vi "PSFL1dll.vi"(8 "error in (no error)":errorcluster, 11 "Inputs":T2) -> (0 "error out":errorcluster, 3 "Outputs":T1)   [LabVIEW 2015]
doc: "SINGLE-PHASE FLASH SUBROUTINES\n\nsubroutine PSFL1dll(p, s, z, kph, t, d, ierr, herr, herr_length)\n\nThese routines accept only single-phase states as inputs. They will be\nfaster than the corresponding general routines, but will fail if called\nwith an incorrect phase specification. The phase-specific subroutines\nalso do not check limits, so may fail if called outside the range of the\nequation of state. The following single-phase routines are available.\n\nINPUTS: \np -- pressure [kPa]\ns -- entropy [[J/mol-K]\nz -- overall (bulk) composition [array of mol frac]\nkph -- phase flag: 1 = liquid\n 2 = vapor\nt -- temperature [K]\nd -- molar density [mol/L]\n\nOUTPUTS:\nt -- temperature [K] (present only for HSFL1)\nd -- molar density [mol/L]\nierr -- error flag: 0 = successful\nherr -- error string (character*255 variable if ierr<>0)\nherr_length -- length of variable herr (default: 255)"
uses:
  REFPROP.dll
panel:
  # "REFPROP-PSFL1dll.vi"
  # "void  PSFL1dll(double *p, double *s, double *z, int32_t *kph, double *t, double *d, int32_t *ierr, CStr herr, int32_t herr_length);"
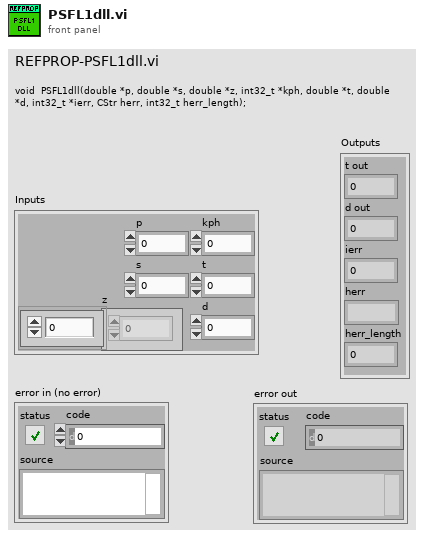
[diagram p1: front panel]
types:
  T1 = cluster{"t out":dbl, "d out":dbl, "ierr":i32, "herr":string, "herr_length":i32}
  T2 = cluster{"p":dbl, "s":dbl, "z":dbl[], "kph":i32, "t":dbl, "d":dbl}
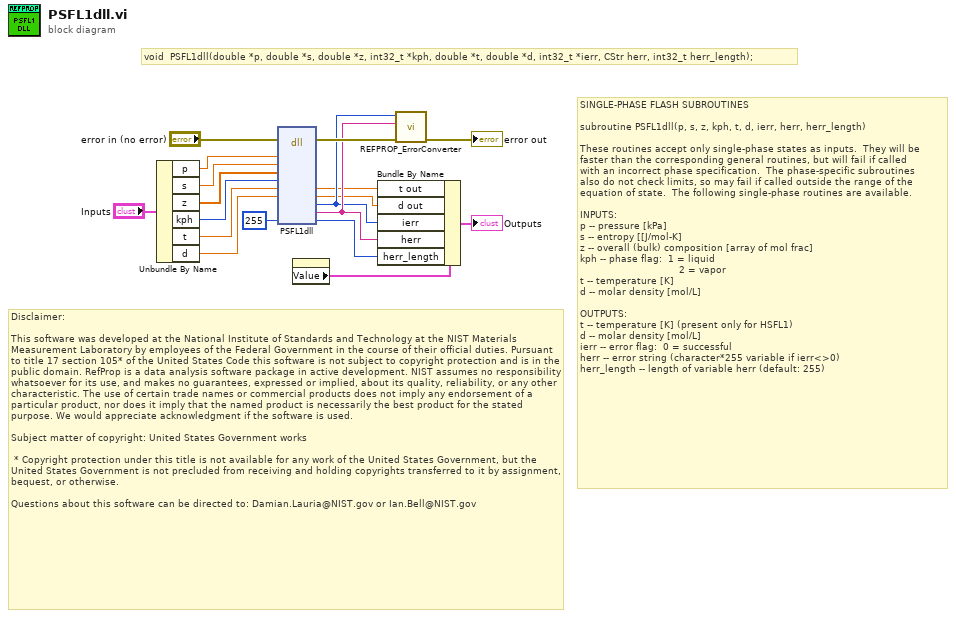
[diagram p0: block diagram]
diagram:
  # "Disclaimer:\n\nThis software was developed at the National Institute of Standards and Technology at the NIST Materials Measurement Laboratory by employees of the Federal Government in the course of their official duties. Pursuant to title 17 section 105* of the United States Code this software is not subject to copyright protection and is in the public domain. RefProp is a data analysis software package in active development. NIST assumes no responsibility whatsoever for its use, and makes no guarantees, expressed or implied, about its quality, reliability, or any other characteristic. The use of certain trade names or commercial products does not imply any endorsement of a particular product, nor does it imply that the named product is necessarily the best product for the stated purpose. We would appreciate acknowledgment if the software is used.\n \nSubject matter of copyright: United States Government works\n  \n * Copyright protection under this title is not available for any work of the United States Government, but the United States Government is not precluded from receiving and holding copyrights transferred to it by assignment, bequest, or otherwise.\n\nQuestions about this software can be directed to: Damian.Lauria@NIST.gov or Ian.Bell@NIST.gov"
  # "void  PSFL1dll(double *p, double *s, double *z, int32_t *kph, double *t, double *d, int32_t *ierr, CStr herr, int32_t herr_length);"
  # "SINGLE-PHASE FLASH SUBROUTINES\n\nsubroutine PSFL1dll(p, s, z, kph, t, d, ierr, herr, herr_length)\n\nThese routines accept only single-phase states as inputs.  They will be\nfaster than the corresponding general routines, but will fail if called\nwith an incorrect phase specification.  The phase-specific subroutines\nalso do not check limits, so may fail if called outside the range of the\nequation of state.  The following single-phase routines are available.\n\nINPUTS: \np -- pressure [kPa]\ns -- entropy [[J/mol-K]\nz -- overall (bulk) composition [array of mol frac]\nkph -- phase flag:  1 = liquid\n                                 2 = vapor\nt -- temperature [K]\nd -- molar density [mol/L]\n\nOUTPUTS:\nt -- temperature [K] (present only for HSFL1)\nd -- molar density [mol/L]\nierr -- error flag:  0 = successful\nherr -- error string (character*255 variable if ierr<>0)\nherr_length -- length of variable herr (default: 255)"
  n1 = Unbundle By Name("Inputs") -> ("p"=w6:dbl, "s"=w5:dbl, "z"=w4:dbl[], "kph"=w3:i32, "t"=w2:dbl, "d"=w1:dbl)
  n2 = dll-call lib="C:/Users/lauria/Desktop/REFPROP 10 LabVIEW Wrapper BETA/REFPROP/REFPROP.*" fn="PSFL1dll"(error in="error in (no error)", "p"=w6, "s"=w5, "z"=w4, "kph"=w3, "t"=w2, "d"=w1, "herr_length"=255) -> (error out=w18:errorcluster, "t"=w8:dbl, "d"=w9:dbl, "ierr"=w10:i32, "herr"=w11:string, "herr_length"=w12:i32)  [unwired: 9 in, 1 out]
  n3 = property on="Outputs" class="Clust (strict)"() -> ("Value"=w14:T1)  [unwired: 2 in, 2 out]
  n4 = Bundle By Name(cluster=w14, "t out"=w8, "d out"=w9, "ierr"=w10, "herr"=w11, "herr_length"=w12) -> (→"Outputs":T1)
  n5 = call "REFPROP_ErrorConverter.vi"("error in (no error)"=w18, "Error Message"=w11, "Error Code"=w10) -> ("error out"=→"error out":errorcluster)  [unwired: 8 in]
